vi "satellite simulator control.vi"() -> ()   [LabVIEW 2012]
uses:
  <vilib>/Utility/error.llb/DialogType.ctl
  <vilib>/DAQmx/create/channels.llb/DAQmx Create Channel (DO-Digital Output).vi
  <vilib>/vision/NI_Vision_Development_Module.lvlib
panel:
  in  "Pixel-Distance Ratio (pix/cm)":dbl=8.26
  in  "Remote Logger Status":bool
  in  "Downlink Object Data?":bool
  in  "Remote Port":u16=61557
  in  "Local Port":u16=61556
  in  "Remote Host":string="localhost"
  in  "broadcast":bool
  in  "Maintain Attitude":bool
  out "alpha":dbl
  out "Objects":T1(array[cluster]) {"Aspect Ratio" format="%.2f"; "Orientation" format="%.2f"; "Area" format="%.2f"; "Object Center"."Y" format="%.2f"; "Object Center"."X" format="%.2f"}
  in  "Y Center Correction":dbl
  in  "X Center Correction":dbl
  out "Offset Degree":dbl
  in  "Y Desired":dbl
  in  "X Desired":dbl
  out "Vx (cm/s)":dbl
  out "Vy (cm/s)":dbl
  in  "OK Button":bool
  out "Filtered Ohmega":dbl
  in  "Air Floating Status":bool
  in  "Control Freq":u32=20
  in  "Alpha Desired":dbl
  in  "STOP":bool caption="stop (F)"
  out "Image Out":T2(plugin-control)
  out "alpha (deg)":dbl
  out "dx (cm)":dbl
  out "dy (cm)":dbl
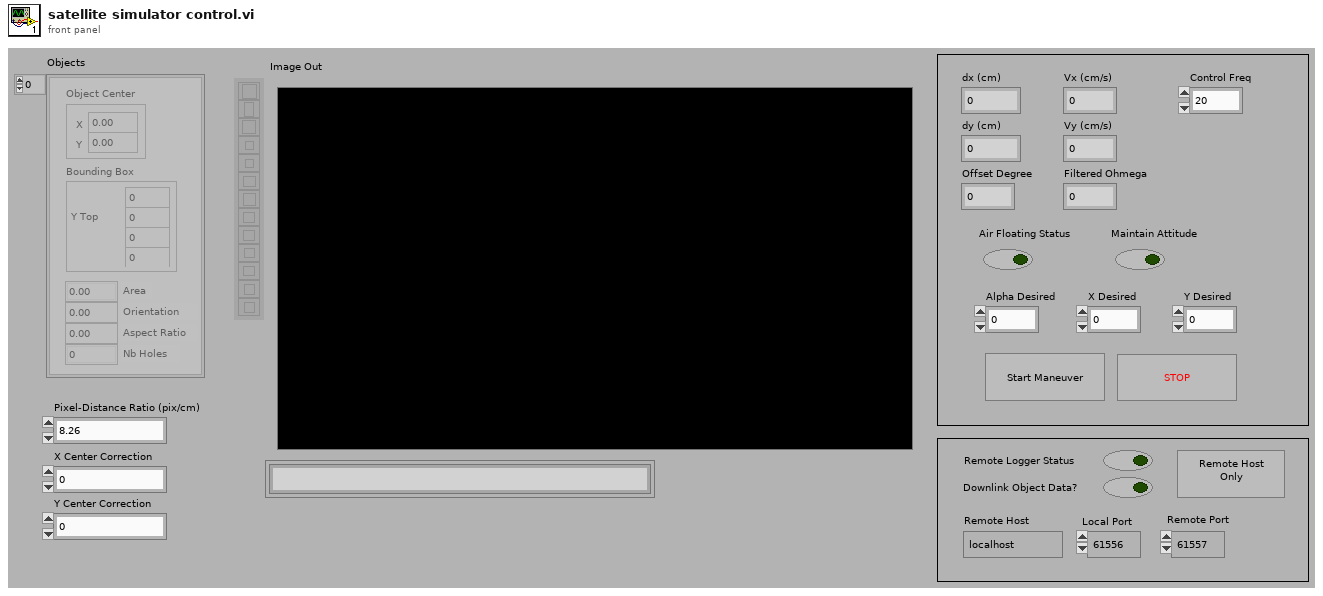
[diagram p1: front panel]
types:
  T1 = cluster{"Object Center":cluster{"X":sgl, "Y":sgl}, "Bounding Box":cluster{"X Left":i32, "Y Top":i32, "X Right":i32, "Y Bottom":i32}, "Area":sgl, "Orientation":sgl, "Aspect Ratio":sgl, "Nb Holes":i32}[]
  T2 = typedef "IMAQ Image.ctl" = refnum<image>
  T3 = typedef "DialogType.ctl" = u16
  T4 = cluster{"dx (cm)":dbl, "dy (cm)":dbl, "Offset Degree":dbl}
  T5 = cluster{"Objects":u16, "Threshold":i32, "Reject Border":bool, "Fill Holes":bool, "Min Object Size":bool, "Min Size":i32, "Max Object Size":bool, "Max Size":i32, "Show Search Area":bool, "Show Center":bool, "Show Bounding Box":bool}
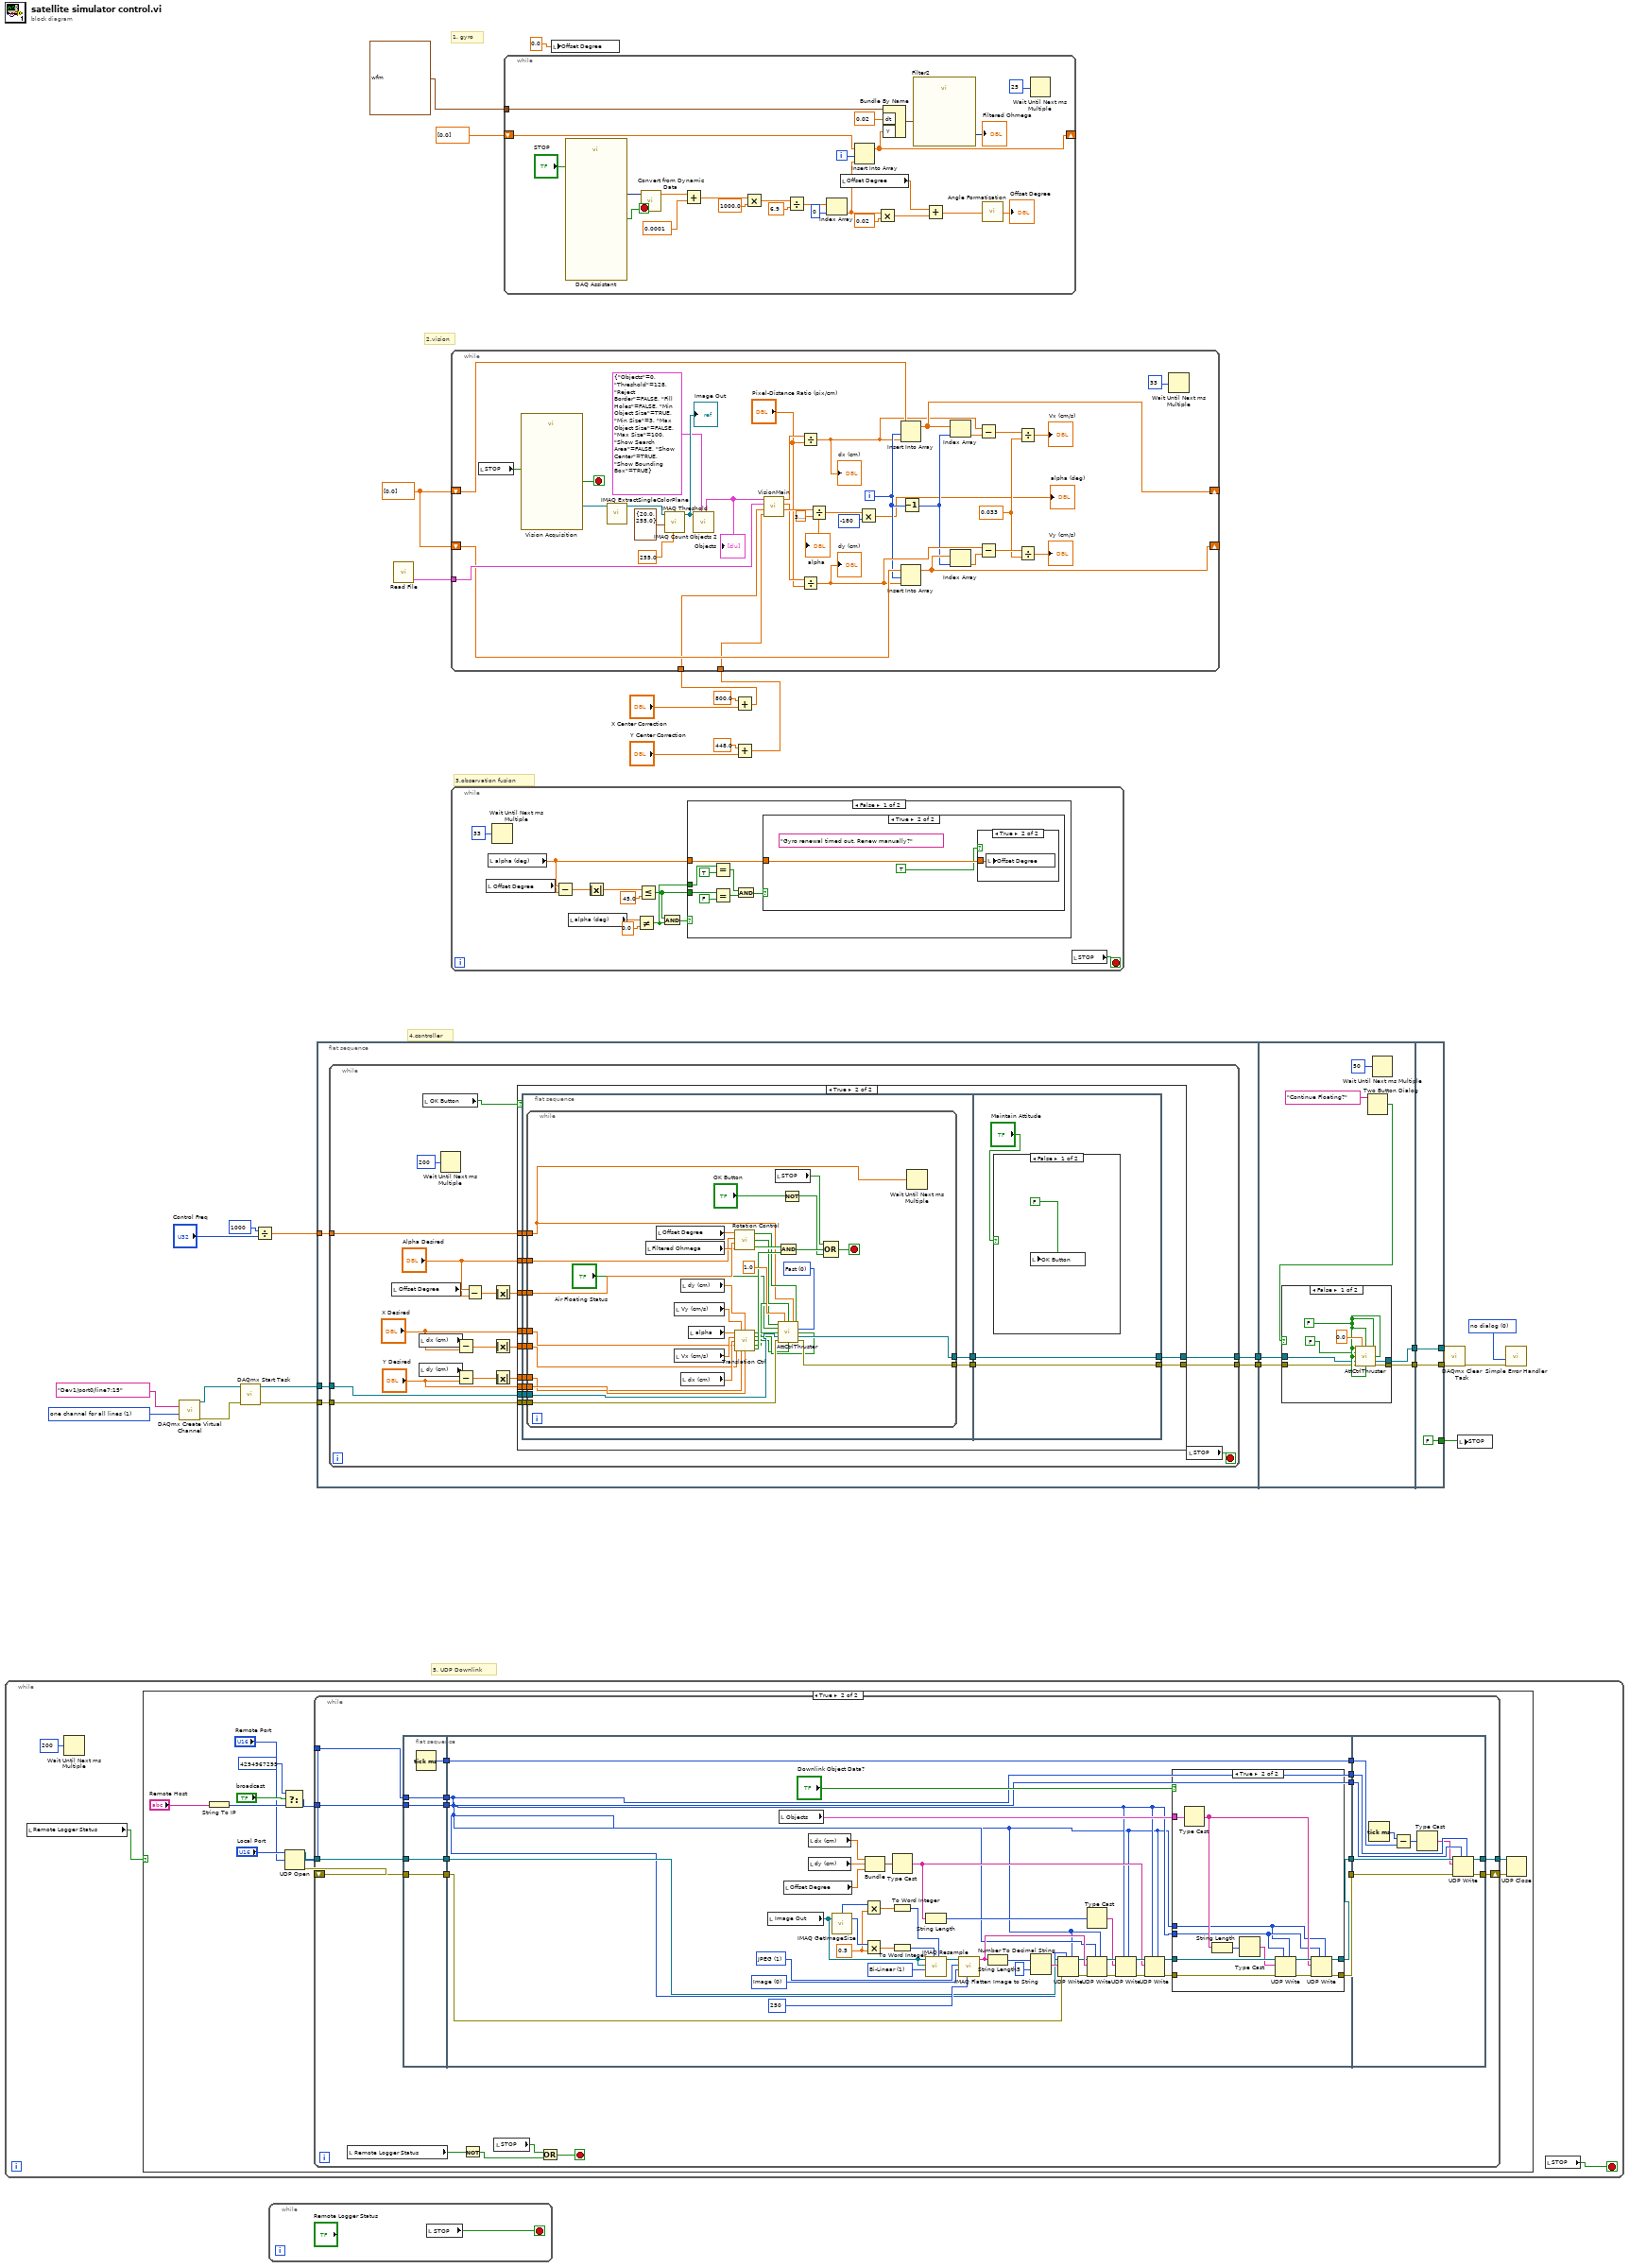
[diagram p0: block diagram]
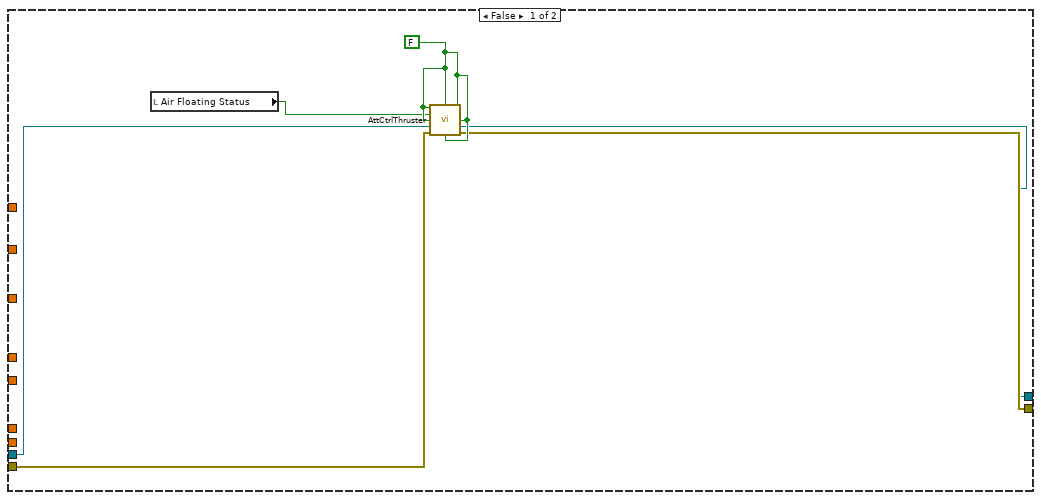
[diagram p4: hidden frame]
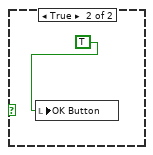
[diagram p5: hidden frame]
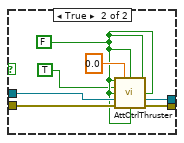
[diagram p6: hidden frame]
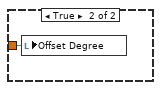
[diagram p9: hidden frame]
diagram:
  w23 = T3 0 items=["no dialog", "OK message", "continue or stop message", "OK message + warnings", "continue/stop + warnings"] ("type of dialog (OK msg:1)")
  w26 = 1 items=["one channel for each line", "one channel for all lines"] ("line grouping")
  w10 = dbl[] [0.0]
  # "5. UDP Downlink"
  # "4.controller"
  # "3.observation fusion"
  # "2.vision"
  # "1. gyro"
  n1 = while {
    stop <- w31 stop-if-true
    n2 = local read "Remote Logger Status"() -> (w32:bool)
    n3 = Wait Until Next ms Multiple(millisecond multiple=u32 200) -> ()  [unwired: 1 out]
    n4 = case shown="True" w32 {
      frame False {
      }
      frame True {
        n5 = String To IP(1:"Remote Host") -> (0:w40:u32)
        n6 = Select(t=u32 4294967295, s="broadcast", f=w40) -> (s? t:f=w37:u32)
        n7 = UDP Open(11:"Local Port") -> (port=w36:refnum<k16>, 0:w35:errorcluster)  [unwired: 1 in, 4 out]
        n8 = while {
          tunnel: "Remote Port" -> [w63]
          tunnel: w37 -> [w62]
          tunnel: w36 -> [w61]
          tunnel: [w59] -> w34
          shift-right: [w58] -> w33
          shift-left: w35 -> [w60]
          stop <- w47 stop-if-true
          n9 = local read "Remote Logger Status"() -> (w45:bool)
          n10 = flat-sequence {
            tunnel: w61 -> [w65]
            tunnel: w63 -> [w66]
            tunnel: w62 -> [w67]
            tunnel: w60 -> [w68]
            tunnel: [w68] -> w57
            tunnel: [w67] -> w56
            tunnel: [w66] -> w55
            tunnel: [w65] -> w54
            tunnel: [w64] -> w53
            tunnel: [w88] -> w52
            tunnel: [w87] -> w51
            tunnel: w57 -> [w106]
            tunnel: w56 -> [w70]
            tunnel: w55 -> [w69]
            tunnel: w54 -> [w90]
            tunnel: [w89] -> w50
            tunnel: w53 -> [w89]
            tunnel: [w69] -> w49
            tunnel: [w70] -> w48
            tunnel: [w130] -> w59
            tunnel: [w124] -> w58
            tunnel: w52 -> [w125]
            tunnel: w51 -> [w131]
            tunnel: w50 -> [w132]
            tunnel: w49 -> [w129]
            tunnel: w48 -> [w128]
            frame #0 {
              n11 = Tick Count (ms)() -> (millisecond timer value=w64:u32)
            }
            frame #1 {
              w94 = u32 1 items=["Zero Order", "Bi-Linear", "Quadratic", "Cubic Spline"] ("Interpolation Type")
              w95 = 0.5
              w103 = 0 items=["Image", "Image and Vision Info", "Reference to Image"] ("Type of Flatten (Image and Vision Info)")
              w108 = 1 items=["None", "JPEG", "PACKED BINARY"] ("Compression (None)")
              n12 = local read "Image Out"() -> (w84:T2)
              n13 = local read "Objects"() -> (w85:T1)
              n14 = local read "Offset Degree"() -> (w81:dbl)
              n15 = local read "dx (cm)"() -> (w83:dbl)
              n16 = local read "dy (cm)"() -> (w82:dbl)
              n17 = call "IMAQ GetImageSize"("Image"=w84) -> ("Y Resolution"=w96:i32, "X Resolution"=w97:i32)  [unwired: 3 in, 1 out]
              n18 = Multiply(x=w97, y=w95) -> (x*y=w99:dbl)
              n19 = Multiply(x=w96, y=w95) -> (x*y=w101:dbl)
              n20 = Bundle("dx (cm)"=w83, "dy (cm)"=w82, "Offset Degree"=w81) -> (w80:T4)  [unwired: 1 in]
              n21 = To Word Integer(number=w99) -> (16bit integer=w98:i16)
              n22 = To Word Integer(number=w101) -> (16bit integer=w100:i16)
              n23 = Type Cast(x=w80) -> (*(type *) &x=w71:string)  [unwired: 1 in]
              n24 = String Length(string=w71) -> (length=w73:i32)
              n25 = call "IMAQ Resample"("X Resolution"=w98, "Y Resolution"=w100, "Interpolation Type"=w94, "Image Dst"=w84, "Image Src"=w84) -> ("Image Dst Out"=w102:T2)  [unwired: 5 in, 1 out]
              n26 = call "IMAQ Flatten Image to String"("Quality (750)"=250, "Type of Flatten (Image and Vision Info)"=w103, "Compression (None)"=w108, "Image"=w102) -> ("Data String"=w107:string)  [unwired: 6 in, 1 out]
              n27 = String Length(string=w107) -> (length=w93:i32)
              n28 = Number To Decimal String(number=w93, width (-)=i16 5) -> (decimal integer string=w92:string)
              n29 = UDP Write(address=w70, port or service name=w69, connection ID=w90, data in=w92, 8:w106) -> (error out=w105:errorcluster, 3:w104:refnum<k16>)  [unwired: 1 out]
              n30 = Type Cast(x=w73) -> (*(type *) &x=w72:string)  [unwired: 1 in]
              n31 = UDP Write(address=w70, port or service name=w69, connection ID=w104, data in=w107, 8:w105) -> (error out=w78:errorcluster, 3:w79:refnum<k16>)  [unwired: 1 out]
              n32 = UDP Write(address=w70, port or service name=w69, connection ID=w79, data in=w72, 8:w78) -> (error out=w77:errorcluster, 3:w75:refnum<k16>)  [unwired: 1 out]
              n33 = UDP Write(address=w70, port or service name=w69, connection ID=w75, data in=w71, 8:w77) -> (error out=w76:errorcluster, 3:w74:refnum<k16>)  [unwired: 1 out]
              n34 = case shown="True" "Downlink Object Data?" {
                tunnel: w85 -> [_ w123]
                tunnel: w76 -> [w111 w121]
                tunnel: [w111 w119] -> w88
                tunnel: w74 -> [w110 w118]
                tunnel: [w110 w116] -> w87
                tunnel: w70 -> [_ w113]
                tunnel: w69 -> [_ w112]
                frame False {
                }
                frame True {
                  n35 = Type Cast(x=w123) -> (*(type *) &x=w114:string)  [unwired: 1 in]
                  n36 = String Length(string=w114) -> (length=w122:i32)
                  n37 = Type Cast(x=w122) -> (*(type *) &x=w115:string)  [unwired: 1 in]
                  n38 = UDP Write(address=w113, port or service name=w112, connection ID=w118, data in=w115, 8:w121) -> (error out=w120:errorcluster, 3:w117:refnum<k16>)  [unwired: 1 out]
                  n39 = UDP Write(address=w113, port or service name=w112, connection ID=w117, data in=w114, 8:w120) -> (error out=w119:errorcluster, 3:w116:refnum<k16>)  [unwired: 1 out]
                }
              }
            }
            frame #2 {
              n40 = Tick Count (ms)() -> (millisecond timer value=w133:u32)
              n41 = Subtract(x=w133, y=w132) -> (x-y=w127:u32)
              n42 = Type Cast(x=w127) -> (*(type *) &x=w126:string)  [unwired: 1 in]
              n43 = UDP Write(address=w128, port or service name=w129, connection ID=w131, data in=w126, 8:w125) -> (error out=w124:errorcluster, 3:w130:refnum<k16>)  [unwired: 1 out]
            }
          }
          n44 = Not(x=w45) -> (.not. x?=w44:bool)
          n45 = local read "STOP"() -> (w46:bool)
          n46 = Or(x=w46, y=w44) -> (x .or. y?=w47:bool)
        }
        n47 = UDP Close(connection ID=w34, 8:w33) -> ()  [unwired: 2 out]
      }
    }
    n48 = local read "STOP"() -> (w31:bool)
  }
  n49 = call-poly <vilib>:"DAQmx Create Virtual Channel.vi"("lines"=tag "Dev1/port0/line7:15" ("Lines"), "line grouping"=w26) -> ("task out"=w24:refnum<k21>, "error out"=w25:errorcluster)  [unwired: 12 in]
  n50 = call <vilib>:"DAQmx Start Task.vi"("task/channels in"=w24, "error in"=w25) -> ("task out"=w19:refnum<k21>, "error out"=w18:errorcluster)  [unwired: 12 in]
  n51 = Divide(x=u32 1000 ("milliseconds to wait"), y="Control Freq") -> (x/y=w15:dbl)
  n52 = while {
    stop <- w134 stop-if-true
    n53 = local read "STOP"() -> (w134:bool)
  }
  n54 = flat-sequence {
    tunnel: w19 -> [w139]
    tunnel: w18 -> [w138]
    tunnel: w15 -> [w135]
    tunnel: [w137] -> w14
    tunnel: [w136] -> w13
    tunnel: w14 -> [w235]
    tunnel: w13 -> [w233]
    tunnel: [w234] -> w3
    tunnel: [w232] -> w2
    tunnel: [w251] -> w16
    tunnel: [w252] -> w17
    tunnel: w3 -> [w252]
    tunnel: w2 -> [w251]
    tunnel: [FALSE] -> w1
    frame #0 {
      n55 = while {
        tunnel: w139 -> [w159]
        tunnel: w138 -> [w158]
        tunnel: [w157] -> w137
        tunnel: [w156] -> w136
        tunnel: w135 -> [w141]
        stop <- w155 stop-if-true
        n56 = local read "Offset Degree"() -> (w154:dbl)
        n57 = local read "dx (cm)"() -> (w150:dbl)
        n58 = local read "dy (cm)"() -> (w146:dbl)
        n59 = local read "OK Button"() -> (w142:bool)
        n60 = Wait Until Next ms Multiple(millisecond multiple=u32 200) -> ()  [unwired: 1 out]
        n61 = Subtract(x=w150, y="X Desired") -> (x-y=w148:dbl)
        n62 = Subtract(x=w146, y="Y Desired") -> (x-y=w144:dbl)
        n63 = Subtract(x=w154, y="Alpha Desired") -> (x-y=w152:dbl)
        n64 = Absolute Value(x=w152) -> (abs(x)=w151:dbl)
        n65 = Absolute Value(x=w148) -> (abs(x)=w147:dbl)
        n66 = Absolute Value(x=w144) -> (abs(x)=w143:dbl)
        n67 = case shown="True" w142 {
          tunnel: w159 -> [w163 w178]
          tunnel: w158 -> [w162 w177]
          tunnel: [w161 w176] -> w157
          tunnel: [w160 w175] -> w156
          tunnel: w141 -> [_ w174]
          tunnel: "Alpha Desired" -> [_ w173]
          tunnel: w151 -> [_ w172]
          tunnel: "X Desired" -> [_ w171]
          tunnel: w147 -> [_ w170]
          tunnel: "Y Desired" -> [_ w169]
          tunnel: w143 -> [_ w168]
          frame False {
            w165 = FALSE
            n68 = local read "Air Floating Status"() -> (w164:bool)
            n69 = call "AttCtrlThruster.vi"("ctclk"=w165, "Up"=w165, "clkwis"=w165, "Float"=w164, "Left"=w165, "Right"=w165, "task in"=w163, "error in"=w162, "Down"=w165) -> ("task out"=w160:refnum<k21>, "error out"=w161:errorcluster)  [unwired: 5 in]
          }
          frame True {
            n70 = flat-sequence {
              tunnel: w178 -> [w189]
              tunnel: w177 -> [w188]
              tunnel: w174 -> [w185]
              tunnel: w173 -> [w184]
              tunnel: w172 -> [w183]
              tunnel: w171 -> [w182]
              tunnel: w170 -> [w181]
              tunnel: w169 -> [w180]
              tunnel: w168 -> [w179]
              tunnel: [w187] -> w167
              tunnel: [w186] -> w166
              tunnel: [w225] -> w175
              tunnel: [w226] -> w176
              tunnel: w167 -> [w226]
              tunnel: w166 -> [w225]
              frame #0 {
                n71 = while {
                  tunnel: w189 -> [w223]
                  tunnel: w188 -> [w222]
                  tunnel: [w220] -> w187
                  tunnel: [w221] -> w186
                  tunnel: w185 -> [w191]
                  tunnel: w184 -> [w201]
                  tunnel: w183 -> [w216]
                  tunnel: w182 -> [w200]
                  tunnel: w181 -> [w211]
                  tunnel: w180 -> [w199]
                  tunnel: w179 -> [w198]
                  stop <- w217 stop-if-true
                  w207 = u16 0 items=["Fast", "Slow"] ("Angular Acceleration")
                  n72 = local read "Filtered Ohmega"() -> (w215:dbl)
                  n73 = local read "Offset Degree"() -> (w214:dbl)
                  n74 = local read "Vy (cm/s)"() -> (w210:dbl)
                  n75 = local read "Vx (cm/s)"() -> (w213:dbl)
                  n76 = local read "dy (cm)"() -> (w209:dbl)
                  n77 = local read "dx (cm)"() -> (w212:dbl)
                  n78 = local read "alpha"() -> (w195:dbl)
                  n79 = call "Rotation Control.vi"("Filtered Ohmega"=w215, "Original Difference"=w216, "Alpha Desired"=w201, "Alpha In"=w214) -> ("Maneuver Complete?"=w194:bool, "Counter-ClkWise Rot Ctrl"=w193:bool, "Clockwise Rot Ctrl"=w192:bool)
                  n80 = call "Translation Ctrl.vi"("Alpha"=w195, "Filtered Speed Y"=w210, "Y In"=w209, "Filtered Speed X"=w213, "X In"=w212, "X Desired"=w200, "Original Difference X"=w211, "Original Difference Y"=w198, "Y Desired"=w199) -> ("Left"=w205:bool, "Right"=w204:bool, "Down"=w203:bool, "Up"=w202:bool, "Maneuver Complete?"=w206:bool)  [unwired: 2 in]
                  n81 = local read "STOP"() -> (w218:bool)
                  n82 = call "AttCtrlThruster.vi"("ctclk"=w193, "Duty Cycle"=1.0, "Up"=w202, "Period"=w191, "clkwis"=w192, "Float"="Air Floating Status", "Angular Acceleration"=w207, "Left"=w205, "Right"=w204, "task in"=w223, "error in"=w222, "Down"=w203) -> ("task out"=w221:refnum<k21>, "error out"=w220:errorcluster)  [unwired: 2 in]
                  n83 = And(x=w194, y=w206) -> (x .and. y?=w208:bool)
                  n84 = Not(x="OK Button") -> (.not. x?=w196:bool)
                  n85 = Compound Arithmetic op=OR(w218, w208, w196) -> (w217:bool)
                  n86 = Wait Until Next ms Multiple(millisecond multiple=w191) -> ()  [unwired: 1 out]
                }
              }
              frame #1 {
                n87 = case shown="False" "Maintain Attitude" {
                  frame False {
                    n88 = local write "OK Button"(FALSE) -> ()
                  }
                  frame True {
                    n89 = local write "OK Button"(TRUE) -> ()
                  }
                }
              }
            }
          }
        }
        n90 = local read "STOP"() -> (w155:bool)
      }
    }
    frame #1 {
      n91 = Two Button Dialog(message="Continue Floating?") -> (T button?=w229:bool)  [unwired: 2 in]
      n92 = case shown="False" w229 {
        tunnel: w235 -> [w238 w249]
        tunnel: [w236 w248] -> w234
        tunnel: w233 -> [w239 w247]
        tunnel: [w237 w246] -> w232
        frame False {
          w241 = FALSE
          n93 = call "AttCtrlThruster.vi"("ctclk"=w241, "Duty Cycle"=0.0, "Up"=w241, "clkwis"=w241, "Float"=FALSE, "Left"=w241, "Right"=w241, "task in"=w239, "error in"=w238, "Down"=w241) -> ("task out"=w237:refnum<k21>, "error out"=w236:errorcluster)  [unwired: 4 in]
        }
        frame True {
          w244 = FALSE
          n94 = call "AttCtrlThruster.vi"("ctclk"=w244, "Duty Cycle"=0.0, "Up"=w244, "clkwis"=w244, "Float"=TRUE, "Left"=w244, "Right"=w244, "task in"=w247, "error in"=w249, "Down"=w244) -> ("task out"=w246:refnum<k21>, "error out"=w248:errorcluster)  [unwired: 4 in]
        }
      }
      n95 = Wait Until Next ms Multiple(millisecond multiple=u32 50) -> ()  [unwired: 1 out]
    }
    frame #2 {
    }
  }
  n96 = call "Read File.vi"() -> ("Objects"=w29:T1)  [unwired: 1 in, 1 out]
  n97 = while {
    stop <- w263 stop-if-true
    n98 = local read "Offset Degree"() -> (w262:dbl)
    n99 = local read "alpha (deg)"() -> (w258:dbl)
    n100 = Wait Until Next ms Multiple(millisecond multiple=u32 33) -> ()  [unwired: 1 out]
    n101 = Subtract(x=w262, y=w258) -> (x-y=w261:dbl)
    n102 = local read "alpha (deg)"() -> (w256:dbl)
    n103 = Absolute Value(x=w261) -> (abs(x)=w260:dbl)
    n104 = Not Equal?(x=w256, y=0.0) -> (x != y?=w254:bool)
    n105 = Less Or Equal?(x=w260, y=45.0) -> (x <= y?=w253:bool)
    n106 = And(x=w253, y=w254) -> (x .and. y?=w257:bool)
    n107 = case shown="False" w257 {
      tunnel: w258 -> [w265 w276]
      tunnel: w254 -> [w267 _]
      tunnel: w253 -> [w266 _]
      frame False {
        n108 = Equal?(x=w267, y=TRUE) -> (x = y?=w271:bool)
        n109 = Equal?(x=w266, y=FALSE) -> (x = y?=w270:bool)
        n110 = And(x=w271, y=w270) -> (x .and. y?=w268:bool)
        n111 = case shown="True" w268 {
          tunnel: w265 -> [_ w274]
          frame False {
          }
          frame True {
            (unwired) "Gyro renewal timed out. Renew manually?" ("message")
            n112 = case shown="True" TRUE {
              tunnel: w274 -> [_ w275]
              frame False {
              }
              frame True {
                n113 = local write "Offset Degree"(w275) -> ()
              }
            }
          }
        }
      }
      frame True {
        n114 = local write "Offset Degree"(w276) -> ()
      }
    }
    n115 = local read "STOP"() -> (w263:bool)
  }
  n116 = while {
    shift-right: [w284] -> _
    shift-left: dbl[] [0.0] -> [w285]
    tunnel: waveform(dbl) {"t0"=timestamp(0 s since 1904-01-01), "dt"=1.0, "Y"=[]} ("waveform") -> [w282]
    i -> [w283]
    stop <- w300 stop-if-true
    n117 = call "DAQ Assistant"("stop (F)"="STOP") -> ("data"=w292:dynamicdata, "stopped"=w300:bool)  [unwired: 15 in, 2 out]
    n118 = call "Convert from Dynamic Data"("Dynamic Data Type"=w292) -> ("Array"=w290:dbl[])  [unwired: 3 in]
    n119 = Add(x=w290, y=0.0001) -> (x+y=w288:dbl[])
    n120 = Multiply(x=w288, y=1000.0) -> (x*y=w299:dbl[])
    n121 = Divide(x=w299, y=6.9) -> (x/y=w293:dbl[])
    n122 = Index Array(array=w293, index=0) -> (element=w278:dbl)
    n123 = local read "Offset Degree"() -> (w287:dbl)
    n124 = Insert Into Array(array=w285, index=w283, new element=w278) -> (w284:dbl[])
    n125 = Multiply(x=w278, y=0.02) -> (x*y=w294:dbl)
    n126 = Bundle By Name(cluster=w282, "dt"=0.02, "Y"=w284) -> (w281:waveform(dbl))
    n127 = call "Filter2"("Signal"=w281) -> ("Filtered Signal"=→"Filtered Ohmega":dynamicdata)  [unwired: 9 in, 1 out]
    n128 = Add(x=w287, y=w294) -> (x+y=w280:dbl)
    n129 = call "Angle Formatization.vi"("Alpha"=w280) -> ("Alpha Formatized"=→"Offset Degree":dbl)
    n130 = Wait Until Next ms Multiple(millisecond multiple=u32 25 ("y")) -> ()  [unwired: 1 out]
  }
  n131 = local write "Offset Degree"(0.0 ("y")) -> ()
  n132 = Add(x=800.0 ("c_x"), y="X Center Correction") -> (x+y=w7:dbl)
  n133 = Add(x=448.0 ("c_y"), y="Y Center Correction") -> (x+y=w4:dbl)
  n134 = while {
    tunnel: w29 -> [w326]
    shift-right: [w323] -> _
    shift-left: w10 -> [w324]
    shift-right: [w312] -> _
    shift-left: w10 -> [w315]
    tunnel: w4 -> [w305]
    tunnel: w7 -> [w304]
    i -> [w314]
    stop <- w337 stop-if-true
    w308 = 0.033 ("y")
    n135 = local read "STOP"() -> (w328:bool)
    n136 = call "Vision Acquisition"("Stop (F)"=w328) -> ("Image Out"=w332:T2, "Stopped"=w337:bool)  [unwired: 24 in, 1 out]
    n137 = call "IMAQ ExtractSingleColorPlane"("Image Src"=w332) -> ("Image Dst Out"=w336:T2)  [unwired: 9 in, 1 out]
    n138 = call "IMAQ Threshold"("Replace Value"=sgl 255.0 ("replace value"), "Range"=cluster{"lower value":sgl, "upper value":sgl} {"lower value"=20.0, "upper value"=255.0} ("threshold"), "Image Src"=w336) -> ("Image Dst Out"=w333:T2)  [unwired: 7 in, 1 out]
    "Image Out" <- w333
    n139 = call "IMAQ Count Objects 2"("Settings"=T5 {"Objects"=0, "Threshold"=128, "Reject Border"=FALSE, "Fill Holes"=FALSE, "Min Object Size"=TRUE, "Min Size"=3, "Max Object Size"=FALSE, "Max Size"=100, "Show Search Area"=FALSE, "Show Center"=TRUE, "Show Bounding Box"=TRUE}, "Image"=w333) -> ("Objects"=w327:T1)  [unwired: 5 in, 4 out]
    "Objects" <- w327
    n140 = call "VisionMain.vi"("Y Center"=w305, "X Center"=w304, "Original Plots"=w326, "Plots Captured"=w327) -> ("alpha"=w325:dbl, "dy"=w321:dbl, "dx"=w316:dbl)  [unwired: 5 in]
    "alpha" <- w325
    n141 = Divide(x=w316, y="Pixel-Distance Ratio (pix/cm)") -> (x/y=w311:dbl)
    "dx (cm)" <- w311
    n142 = Divide(x=w321, y="Pixel-Distance Ratio (pix/cm)") -> (x/y=w320:dbl)
    "dy (cm)" <- w320
    n143 = Divide(x=w325, y=3.141592653589793) -> (x/y=w330:dbl)
    n144 = Multiply(x=w330, y=-180) -> (x*y=→"alpha (deg)":dbl)
    n145 = Insert Into Array(array=w315, index=w314, new element=w311) -> (w312:dbl[])
    n146 = Insert Into Array(array=w324, index=w314, new element=w320) -> (w323:dbl[])
    n147 = Decrement(x=w314) -> (x-1=w313:i32)
    n148 = Index Array(array=w312, index=w313) -> (element=w310:dbl)
    n149 = Index Array(array=w323, index=w313) -> (element=w322:dbl)
    n150 = Subtract(x=w311, y=w310) -> (x-y=w309:dbl)
    n151 = Subtract(x=w320, y=w322) -> (x-y=w319:dbl)
    n152 = Divide(x=w309, y=w308) -> (x/y=→"Vx (cm/s)":dbl)
    n153 = Divide(x=w319, y=w308) -> (x/y=→"Vy (cm/s)":dbl)
    n154 = Wait Until Next ms Multiple(millisecond multiple=u32 33) -> ()  [unwired: 1 out]
  }
  n155 = call <vilib>:"DAQmx Clear Task.vi"("task in"=w16, "error in"=w17) -> ("error out"=w22:errorcluster)  [unwired: 13 in]
  n156 = local write "STOP"(w1) -> ()
  n157 = call <vilib>:"Simple Error Handler.vi"("type of dialog (OK msg:1)"=w23, "error in (no error)"=w22) -> ()  [unwired: 3 in, 5 out]
